vi "Remove Page Attachments.vi"(7 "Atlassian Connection in":refnum<class "Confluence.lvclass">, 8 "Error in":errorcluster caption="Error in (no error)", 11 "Page in":refnum<class "Page.lvclass">) -> (0 "Error out":errorcluster, 2 "# Attachments Removed":i32, 3 "Page out":refnum<class "Page.lvclass">, 5 "Atlassian Connection out":refnum<class "Confluence.lvclass">)   [LabVIEW 2023, in "VIDoc Printer - Confluence.lvlib" / "VIDoc Printer - Confluence.lvclass"]
uses:
  VIDoc Printer - Confluence.lvclass
  VIDoc Printer - Confluence.lvclass/VIDoc Printer - Confluence.ctl
  <userlib>/_PetranWay/LabVIEW Confluence API/Source/Confluence/Page/Page.lvclass
  <userlib>/_PetranWay/LabVIEW Confluence API/Source/Confluence/Confluence Connection/Confluence.lvclass
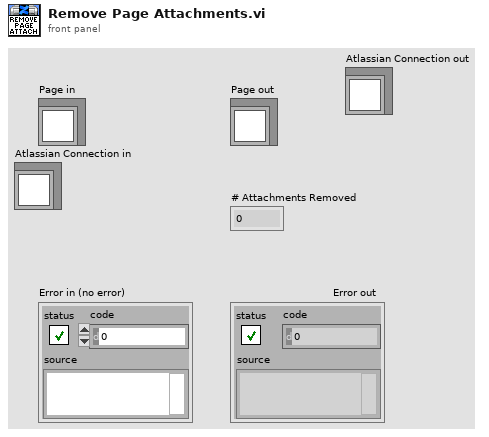
[diagram p1: front panel]
types:
  T1 = typedef "PetranWay_Confluence API.lvlib/Page.lvclass/Attachment Information.ctl" = cluster{"id":string, "type":string, "status":string, "<UTF8>title":string, "version":cluster{"number":dbl}}
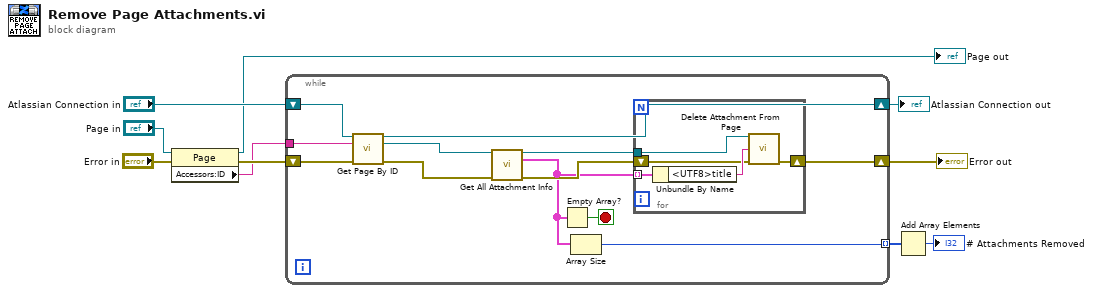
[diagram p0: block diagram]
diagram:
  n1 = property on="Property Node" class="Page"(reference="Page in", error in="Error in") -> (reference out=→"Page out":refnum<class "Page.lvclass">, error out=w10:errorcluster, "Accessors:ID"=w9:string)
  n2 = while {
    shift-right: [w22] -> w3
    shift-left: "Atlassian Connection in" -> [w21]
    shift-right: [w18] -> w4
    shift-left: w10 -> [w19]
    tunnel: w9 -> [w17]
    tunnel: [w16] -> w6 mode=indexing
    stop <- w20 stop-if-true
    n3 = call-dynamic "Get Page By ID.vi"("Confluence Connection in"=w21, "ID"=w17, "error in (no error)"=w19) -> ("Atlassian Connection out"=w22:refnum<class "Confluence.lvclass">, "Page out"=w15:refnum<class "Page.lvclass">, "error out"=w14:errorcluster)  [unwired: 9 in, 1 out]
    n4 = call-dynamic "Get All Attachment Info.vi"("Page in"=w15, "error in (no error)"=w14) -> ("Page out"=w12:refnum<class "Page.lvclass">, "Attachement Information"=w11:T1[], "error out"=w13:errorcluster)  [unwired: 10 in, 1 out]
    n5 = Empty Array?(array=w11) -> (empty?=w20:bool)
    n6 = Array Size(array=w11) -> (size(s)=w16:i32)
    n7 = for {
      tunnel: w11 -> [w27] mode=indexing
      shift-right: [w24] -> w18
      shift-left: w13 -> [w25]
      tunnel: w12 -> [w23]
      n8 = Unbundle By Name(w27) -> ("<UTF8>title"=w26:string)
      n9 = call-dynamic "Delete Attachment From Page.vi"("Page"=w23, "Attachment File Name to Delete"=w26, "error in (no error)"=w25) -> ("error out"=w24:errorcluster)  [unwired: 11 in, 1 out]
    }
  }
  "Error out" <- w4
  "Atlassian Connection out" <- w3
  n10 = Add Array Elements(numeric array=w6) -> (sum=→"# Attachments Removed":i32)
